vi "Get Settings.vi"(8 "error in (no error)":errorcluster, 11 "Application in":refnum<class "Application.lvclass">) -> (0 "error out":errorcluster, 2 "Settings":T1, 3 "Application out":refnum<class "Application.lvclass">)   [LabVIEW 2019, in "Application.lvclass"]
doc: "Developed by Kevin Thompson\nkevin@thompsonengineering.net\n\nCopyright 2018\nThompson Engineering, LLC"
uses:
  Application.lvclass
  DataTypes/Settings--cluster.ctl
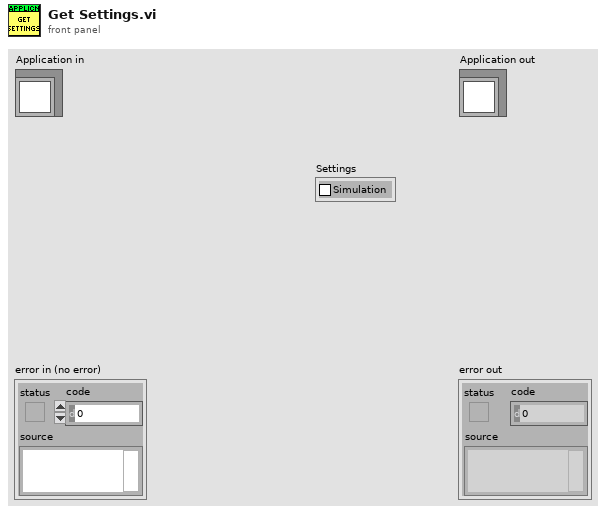
[diagram p1: front panel]
types:
  T1 = typedef "Application.lvclass/Settings--cluster.ctl" = cluster{"Simulation":bool}
  T2 = typedef "Application.lvclass/ObjData--cluster.ctl" = cluster{"Settings":T1, "Public Events":T3, "Dependency":T4, "ReadData-placeholder":T5, "VISA-placeholder":refnum<visa-resource-name>, "Subsys ClassRefs Dict":T6, "InverterWaveformsQ":T7, "RawDaqDataQ":T8}
  T3 = typedef "Application.lvclass/Public Events--cluster.ctl" = cluster{"Application.AsyncCmd Event":refnum<user-event>, "Application.AsyncMsg Event":refnum<user-event>, "stop process":refnum<user-event>}
  T4 = typedef "Application.lvclass/Dependency--cluster.ctl" = cluster{"Config":refnum<class "Config.lvclass">, "Main":refnum<class "Main.lvclass">, "ErrorHandler":refnum<class "ErrorHandler.lvclass">, "DAQ_Engine":refnum<class "DAQ_Engine.lvclass">, "Log_Engine":refnum<class "Log_Engine.lvclass">}
  T5 = typedef "Application.lvclass/Read Data--cluster.ctl" = cluster{"Data":dbl}
  T6 = typedef "TD Dynamic CVT DVR--ref.ctl" = refnum<data-value>
  T7 = typedef "InverterWaveforms--QRef.ctl" = refnum<queue>
  T8 = typedef "RawDAQDataQRef--cluster.ctl" = refnum<queue>
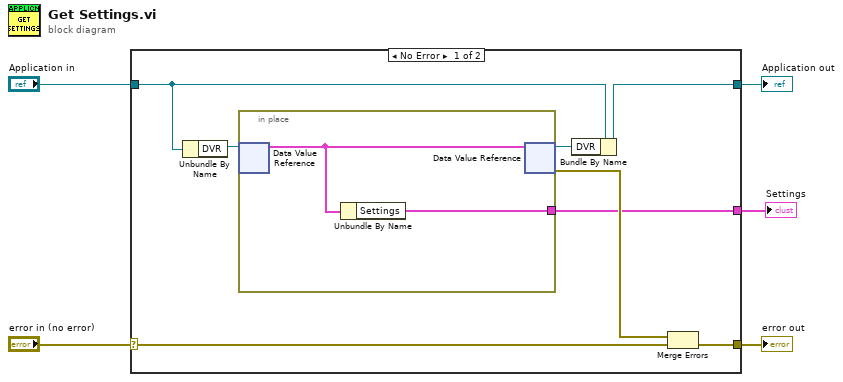
[diagram p0: block diagram]
diagram:
  n1 = case shown="No Error" "error in (no error)" {
    selector: "error in (no error)" -> [w13 w16]
    tunnel: [w8 w16] -> w4
    tunnel: [w9 w17] -> w2
    tunnel: "Application in" -> [w10 w17]
    tunnel: [w6 _] -> w1
    frame No Error {
      n2 = Unbundle By Name(w10) -> ("DVR"=w11:refnum<data-value>)
      n3 = in-place {
        in-place-border: [w14] -> w6
        n4 = in-place-dvr #1(w11) -> (w15:T2)  [unwired: 1 out]
        n5 = Unbundle By Name(w15) -> ("Settings"=w14:T1)
        n6 = in-place-dvr #1(w15) -> (w12:refnum<data-value>, w7:errorcluster)
      }
      n7 = Bundle By Name(cluster=w10, "DVR"=w12) -> (w9:refnum<class "Application.lvclass">)
      n8 = Merge Errors(w7, w13) -> (w8:errorcluster)
    }
    frame Error {
    }
  }
  "error out" <- w4
  "Application out" <- w2
  "Settings" <- w1
